vi "calNormalize.vi"(4 "532 pd Cal":dbl=0.79, 6 "660 pd Cal":dbl=1.53, 10 "pd data":cluster{dbl[][], dbl[][]}, 11 "mic data":cluster{dbl[][], dbl[][]}) -> (2 "660 Normalized":dbl[](array[numeric]), 3 "532 Normalized":dbl[](array[numeric]))   [LabVIEW 2011]
uses:
  <vilib>/Analysis/NI_AALBase.lvlib
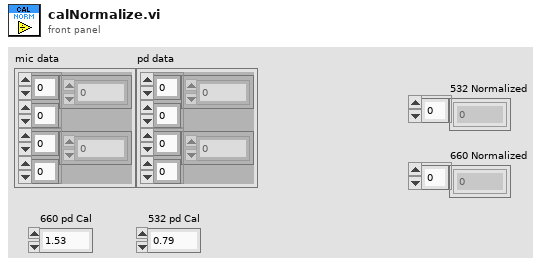
[diagram p1: front panel]
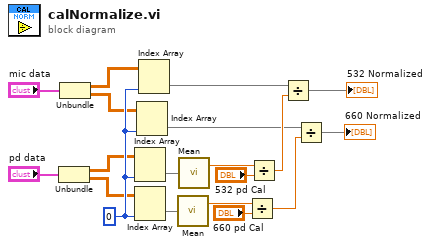
[diagram p0: block diagram]
diagram:
  w9 = 0 ("disabled index (col)")
  n1 = Unbundle("pd data") -> (w5:dbl[][], w4:dbl[][])
  n2 = Unbundle("mic data") -> (w7:dbl[][], w6:dbl[][])
  n3 = Index Array(array=w5, index (col)=w9) -> (element=w2:dbl[])  [unwired: 1 in]
  n4 = Index Array(array=w4, index (col)=w9) -> (element=w1:dbl[])  [unwired: 1 in]
  n5 = Index Array(array=w6, index (col)=w9) -> (element=w11:dbl[])  [unwired: 1 in]
  n6 = Index Array(array=w7, index (col)=w9) -> (element=w10:dbl[])  [unwired: 1 in]
  n7 = call <vilib>:"Mean.vi"("X"=w1) -> ("mean"=w14:dbl)  [unwired: 1 out]
  n8 = call <vilib>:"Mean.vi"("X"=w2) -> ("mean"=w18:dbl)  [unwired: 1 out]
  n9 = Divide(x=w14, y="660 pd Cal") -> (x/y=w16:dbl)
  n10 = Divide(x=w18, y="532 pd Cal") -> (x/y=w19:dbl)
  n11 = Divide(x=w10, y=w19) -> (x/y=→"532 Normalized":dbl[])
  n12 = Divide(x=w11, y=w16) -> (x/y=→"660 Normalized":dbl[])
